vi "Start all 4 Axis Movement.vi"(4 "error in (no error)":errorcluster, 7 "Mint Controller reference":refnum<k7>) -> (0 "error out":errorcluster, 3 "Mint Controller reference out":refnum<k7>)   [LabVIEW 2015]
doc: "Triggers all 4 axis to stat the movement to thier target positions."
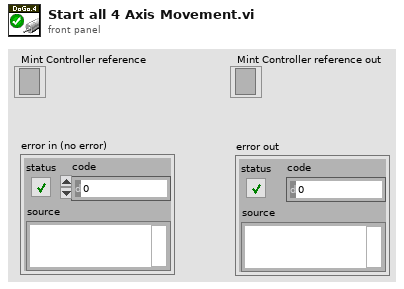
[diagram p1: front panel]
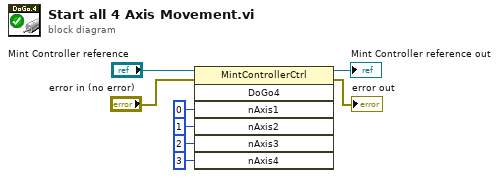
[diagram p0: block diagram]
diagram:
  n1 = invoke class="MintControllerCtrl" method="DoGo4"(reference="Mint Controller reference", error in="error in (no error)", "nAxis1"=i16 0, "nAxis2"=i16 1, "nAxis3"=i16 2, "nAxis4"=i16 3) -> (reference out=→"Mint Controller reference out":refnum<k7>, error out=→"error out":errorcluster)  [unwired: 1 in, 5 out]
